vi "LBCB Position Facade.vi"(0 "Data In":T6, 2 "Display State In":T3, 3 "Container State":T5) -> (6 "Data Out":T6, 7 "Display State Out":T3, 8 "Action":T2)   [LabVIEW 2013, in "LBCB Position XC.xctl"]
uses:
  LBCB Position XC.xctl
  lib/Data Access Objects/Metadata/LBCB Position.ctl
  LBCB Position Data.ctl
  <vilib>/_xctls/Container State.ctl
  LBCB Position State.ctl
  lib/Data Access Objects/Application/Number Of LBCBs.ctl
  <vilib>/_xctls/Action.ctl
  <vilib>/_xctls/XControlSupport.lvlib
panel:
  in  "LBCB Position Tab":enum32{"LBCB 1", "LBCB 2"}(tab)
  in  "LBCB Position L1":T1={"Motion Center"=[0.0, 0.0, 0.0], "Transformation Matrix"=[[1.0, 0.0, 0.0, 0.0, 0.0, 0.0], [0.0, 1.0, 0.0, 0.0, 0.0, 0.0], [0.0, 0.0, 1.0, 0.0, 0.0, 0.0], [0.0, 0.0, 0.0, 1.0, 0.0, 0.0], [0.0, 0.0, 0.0, 0.0, 1.0, 0.0], [0.0, 0.0, 0.0, 0.0, 0.0, 1.0]]}
  in  "LBCB Position L2":T1={"Motion Center"=[0.0, 0.0, 0.0], "Transformation Matrix"=[[1.0, 0.0, 0.0, 0.0, 0.0, 0.0], [0.0, 1.0, 0.0, 0.0, 0.0, 0.0], [0.0, 0.0, 1.0, 0.0, 0.0, 0.0], [0.0, 0.0, 0.0, 1.0, 0.0, 0.0], [0.0, 0.0, 0.0, 0.0, 1.0, 0.0], [0.0, 0.0, 0.0, 0.0, 0.0, 1.0]]}
  # "Y"
  # "X"
  # "(inch)"
  # "XLBCB CMD = T-1*XLBCB OM"
  # "Y"
  # "Z"
  # "(inch)"
  # "XOM DISP = T*XLBCB DISP"
  # "Z"
  # "(inch)"
  # "Dx"
  # "Dy"
  # "Dz"
  # "Rx"
  # "Ry"
  # "Rz"
  # "Dx"
  # "Dy"
  # "Dz"
  # "Rx"
  # "Ry"
  # "Rz"
  # "Y"
  # "X"
  # "(inch)"
  # "XLBCB CMD = T-1*XLBCB OM"
  # "Y"
  # "Z"
  # "(inch)"
  # "XOM DISP = T*XLBCB DISP"
  # "Z"
  # "(inch)"
  # "Dx"
  # "Dy"
  # "Dz"
  # "Rx"
  # "Ry"
  # "Rz"
  # "Dx"
  # "Dy"
  # "Dz"
  # "Rx"
  # "Ry"
  # "Rz"
  # "Y"
  # "X"
  # "(inch)"
  # "XLBCB CMD = T-1*XLBCB OM"
  # "Y"
  # "Z"
  # "(inch)"
  # "XOM DISP = T*XLBCB DISP"
  # "Z"
  # "(inch)"
  # "Dx"
  # "Dy"
  # "Dz"
  # "Rx"
  # "Ry"
  # "Rz"
  # "Dx"
  # "Dy"
  # "Dz"
  # "Rx"
  # "Ry"
  # "Rz"
  # "Y"
  # "X"
  # "(inch)"
  # "XLBCB CMD = T-1*XLBCB OM"
  # "Y"
  # "Z"
  # "(inch)"
  # "XOM DISP = T*XLBCB DISP"
  # "Z"
  # "(inch)"
  # "Dx"
  # "Dy"
  # "Dz"
  # "Rx"
  # "Ry"
  # "Rz"
  # "Dx"
  # "Dy"
  # "Dz"
  # "Rx"
  # "Ry"
  # "Rz"
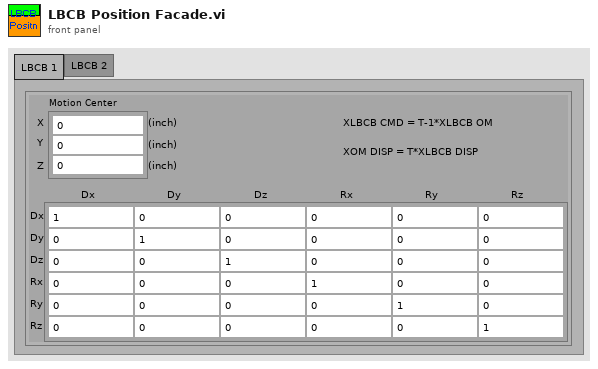
[diagram p1: front panel]
types:
  T1 = typedef "LBCB Position.ctl" = cluster{"Motion Center":dbl[], "Transformation Matrix":dbl[][]}
  T2 = typedef "XControlSupport.lvlib/Action.ctl" = cluster{"Data Changed?":bool, "State Changed?":bool, "Action Name":string}
  T3 = typedef "LBCB Position XC.xctl/LBCB Position State.ctl" = cluster{"Number of LBCBs":T4}
  T4 = typedef "Number Of LBCBs.ctl" = enum16{"1", "2"}
  T5 = typedef "XControlSupport.lvlib/Container State.ctl" = cluster{"Indicator?":bool, "Run Mode?":bool, " Refnum":refnum<vi>}
  T6 = typedef "LBCB Position XC.xctl/LBCB Position Data.ctl" = cluster{"Motion Center":dbl[], "Transformation Matrix":dbl[][]}[]
  T7 = enum8{"Enabled", "Disabled", "Disabled and Grayed Out"}
  T8 = cluster{"Motion Center":dbl[], "Transformation Matrix":dbl[][]}
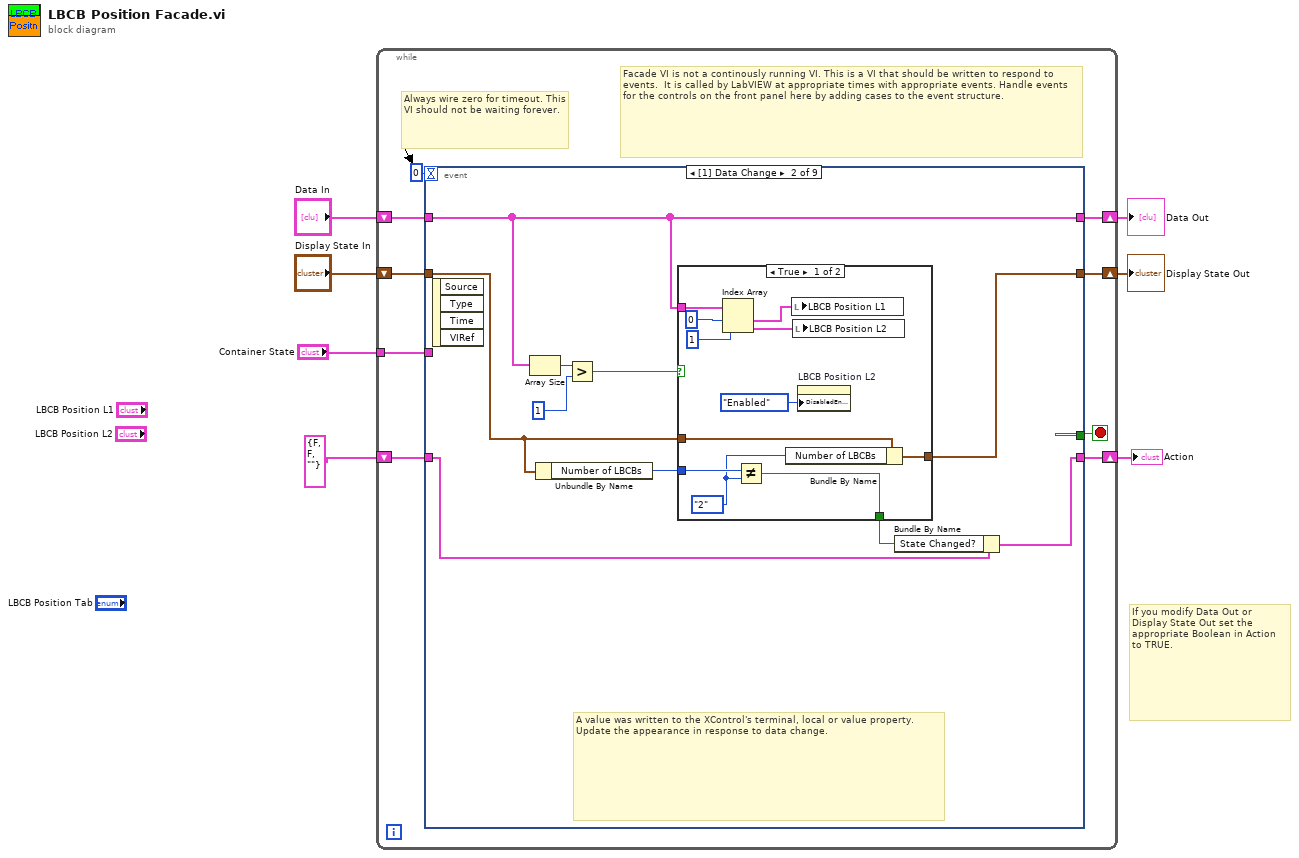
[diagram p0: block diagram]
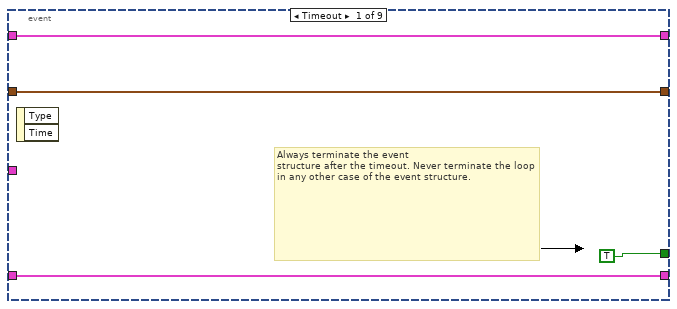
[diagram p2: hidden frame]
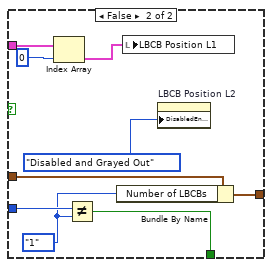
[diagram p3: hidden frame]
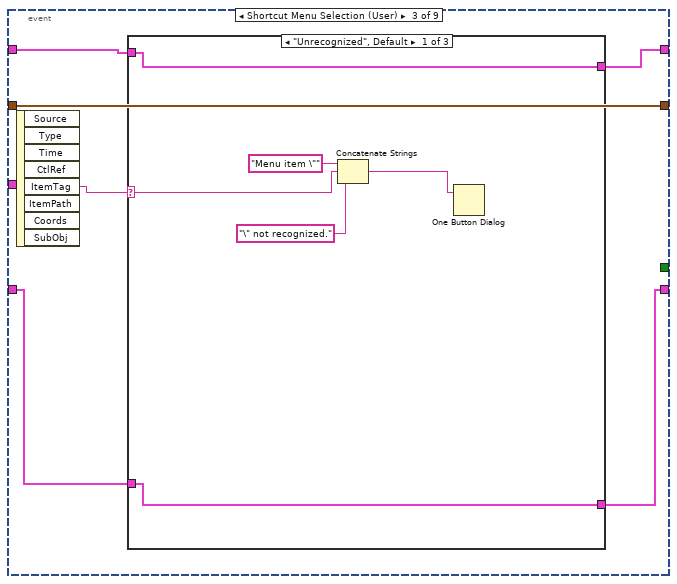
[diagram p4: hidden frame]
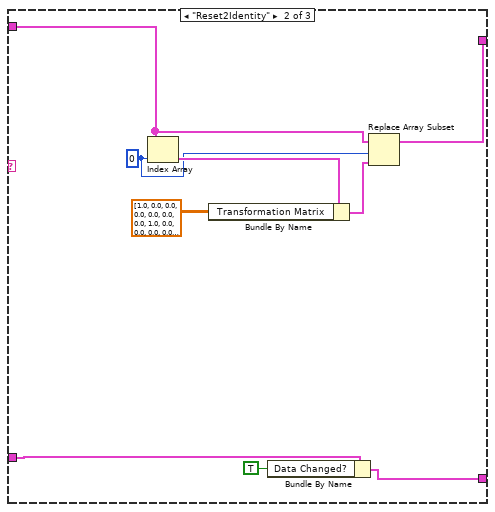
[diagram p5: hidden frame]
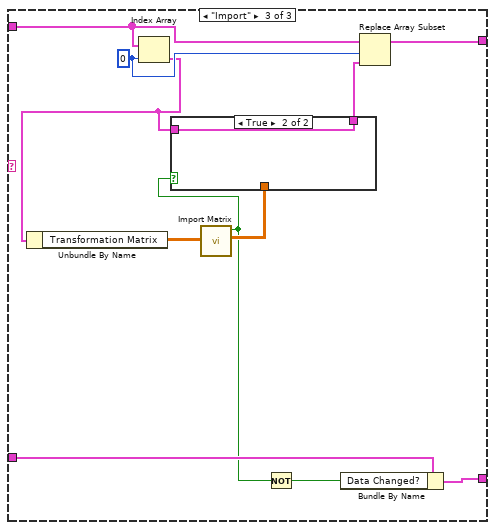
[diagram p6: hidden frame]
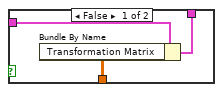
[diagram p7: hidden frame]
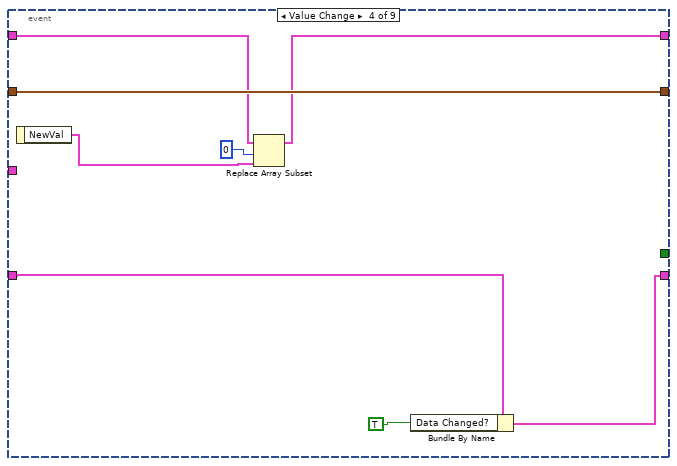
[diagram p8: hidden frame]
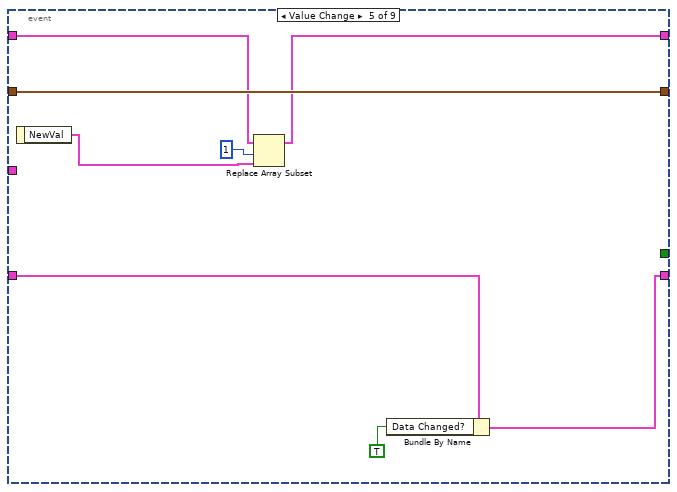
[diagram p9: hidden frame]
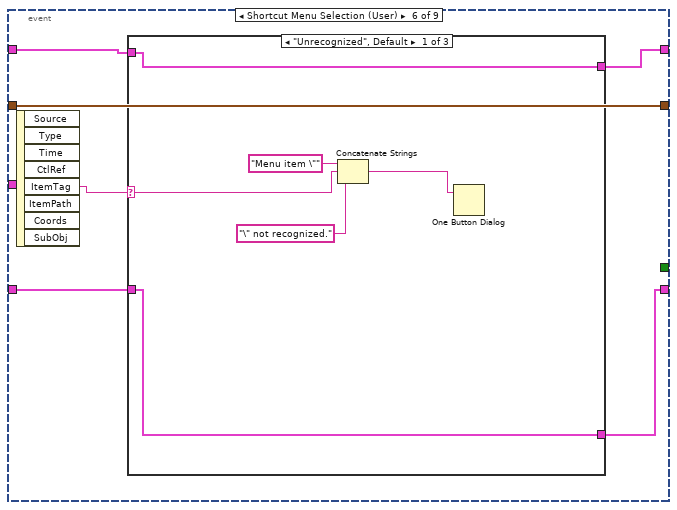
[diagram p10: hidden frame]
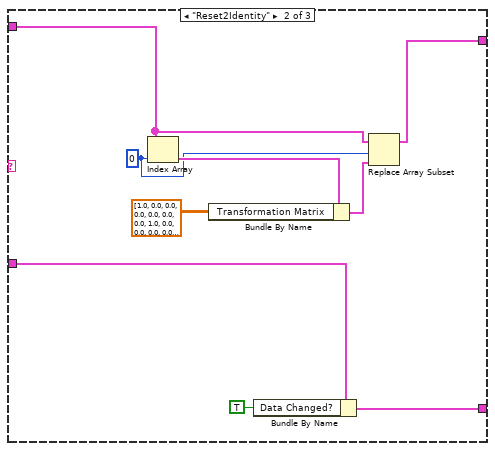
[diagram p11: hidden frame]
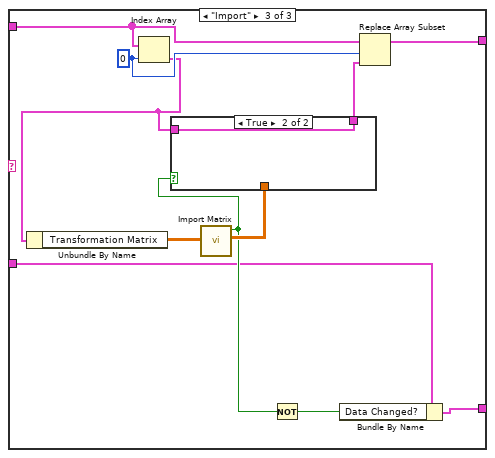
[diagram p12: hidden frame]
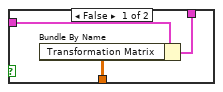
[diagram p13: hidden frame]
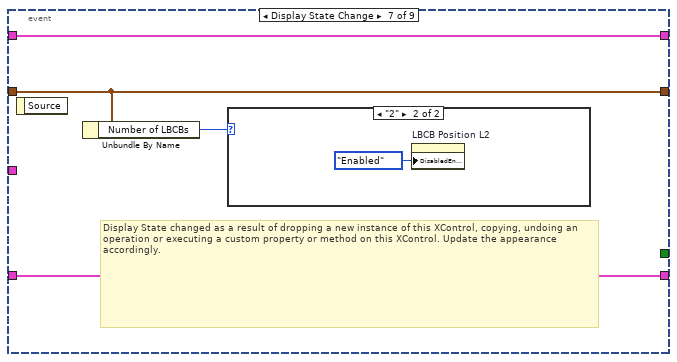
[diagram p14: hidden frame]
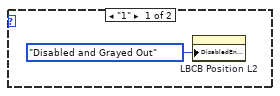
[diagram p15: hidden frame]
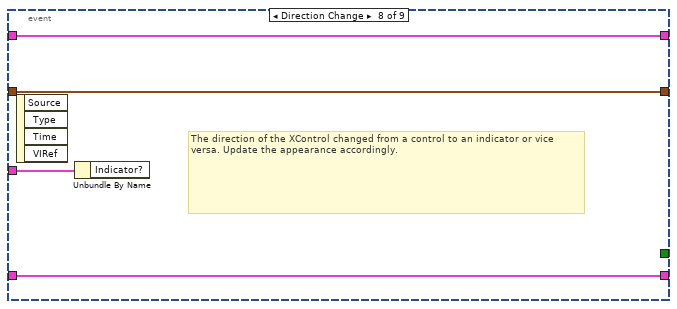
[diagram p16: hidden frame]
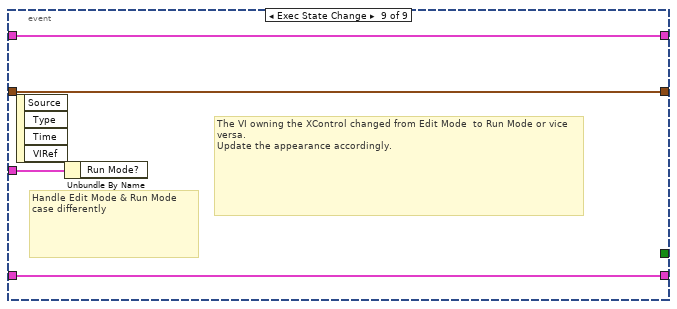
[diagram p17: hidden frame]
diagram:
  # "If you modify Data Out or\nDisplay State Out set the\nappropriate Boolean in Action\nto TRUE."
  n1 = while {
    shift-right: [w15] -> w4
    shift-left: "Display State In" -> [w16]
    tunnel: "Container State" -> [w12]
    shift-right: [w10] -> w7
    shift-left: "Data In" -> [w11]
    shift-right: [w8] -> w2
    shift-left: T2 {"Data Changed?"=FALSE, "State Changed?"=FALSE, "Action Name"=""} ("Action") -> [w9]
    stop <- w14 stop-if-true
    # "Facade VI is not a continously running VI. This is a VI that should be written to respond to events.  It is called by LabVIEW at appropriate times with appropriate events. Handle events for the controls on the front panel here by adding cases to the event structure."
    # "Always wire zero for timeout. This\nVI should not be waiting forever."
    n2 = event shown="[1] Data Change" {
      selector: _ -> [_ _ _ _ _ _ _ _ _]
      dyn-events: _ -> [_ _ _ _ _ _ _ _ _]
      timeout: 0 -> [_ _ _ _ _ _ _ _ _]
      tunnel: w16 -> [w18 w26 w56 w94 w102 w108 w140 w147 w151]
      tunnel: [w18 w21 w56 w94 w102 w108 w140 w147 w151] -> w15
      tunnel: [TRUE _ _ _ _ _ _ _ _] -> w14
      tunnel: w12 -> [_ _ _ _ _ _ _ w148 w152]
      tunnel: w11 -> [w17 w30 w54 w93 w101 w106 w142 w146 w150]
      tunnel: [w17 w30 w53 w90 w98 w105 w142 w146 w150] -> w10
      tunnel: [w19 w22 w51 w88 w95 w103 w141 w145 w149] -> w8
      tunnel: w9 -> [w19 w23 w52 w89 w96 w104 w141 w145 w149]
      event Timeout {
        # "Always terminate the event\nstructure after the timeout. Never terminate the loop in any other case of the event structure."
        n3 = event-data() -> ()  [unwired: 1 in, 2 out]
      }
      event Data Change {
        # "A value was written to the XControl's terminal, local or value property.\nUpdate the appearance in response to data change."
        n4 = event-data() -> ()  [unwired: 1 in, 4 out]
        n5 = Array Size(array=w30) -> (size(s)=w29:i32)
        n6 = Unbundle By Name(w26) -> ("Number of LBCBs"=w25:T4)
        n7 = Greater?(x=w29, y=1) -> (0:w27:bool)
        n8 = case shown="True" w27 {
          tunnel: w30 -> [w41 w50]
          tunnel: w26 -> [w34 w45]
          tunnel: w25 -> [w35 w46]
          tunnel: [w32 w43] -> w24
          tunnel: [w31 w42] -> w21
          frame True {
            w33 = Number_Of_LBCBs."2" ("y")
            n9 = Index Array(array=w41, index #1=0 ("index"), index #2=1 ("index")) -> (element #1=w38:T8, element #2=w37:T8)
            n10 = Not Equal?(x=w35, y=w33) -> (x != y?=w32:bool)
            n11 = Bundle By Name(cluster=w34, "Number of LBCBs"=w33) -> (w31:T3)
            n12 = local write "LBCB Position L1"(w38) -> ()
            n13 = local write "LBCB Position L2"(w37) -> ()
            n14 = property on="LBCB Position L2" class="Clust (strict)"("DisabledEnum"=T7."Enabled" ("Disabled")) -> ()  [unwired: 2 in, 2 out]
          }
          frame False {
            w44 = Number_Of_LBCBs."1" ("y")
            n15 = Index Array(array=w50, index=0) -> (element=w48:T8)
            n16 = Not Equal?(x=w46, y=w44) -> (x != y?=w43:bool)
            n17 = Bundle By Name(cluster=w45, "Number of LBCBs"=w44) -> (w42:T3)
            n18 = local write "LBCB Position L1"(w48) -> ()
            n19 = property on="LBCB Position L2" class="Clust (strict)"("DisabledEnum"=T7."Disabled and Grayed Out" ("Disabled")) -> ()  [unwired: 2 in, 2 out]
          }
        }
        n20 = Bundle By Name(cluster=w23, "State Changed?"=w24) -> (w22:T2)
      }
      event Shortcut Menu Selection (User) {
        n21 = event-data() -> ("ItemTag"=w55:string)  [unwired: 1 in, 7 out]
        n22 = case shown="\"Unrecognized\", Default" w55 {
          selector: w55 -> [w60 _ _]
          tunnel: w54 -> [w58 w68 w81]
          tunnel: [w58 w66 w79] -> w53
          tunnel: w52 -> [w57 w65 w75]
          tunnel: [w57 w64 w74] -> w51
          frame "Unrecognized", Default {
            n23 = Concatenate Strings("Menu item \"" ("string"), w60, "\" not recognized." ("string")) -> (w59:string)
            n24 = One Button Dialog(message=w59) -> ()  [unwired: 1 in, 1 out]
          }
          frame "Reset2Identity" {
            w69 = 0 ("index")
            n25 = Index Array(array=w68, index=w69) -> (element=w71:T8)
            n26 = Bundle By Name(cluster=w71, "Transformation Matrix"=dbl[][] [[1.0, 0.0, 0.0, 0.0, 0.0, 0.0], [0.0, 1.0, 0.0, 0.0, 0.0, 0.0], [0.0, 0.0, 1.0, 0.0, 0.0, 0.0], [0.0, 0.0, 0.0, 1.0, 0.0, 0.0], [0.0, 0.0, 0.0, 0.0, 1.0, 0.0], [0.0, 0.0, 0.0, 0.0, 0.0, 1.0]]) -> (w67:T8)
            n27 = Bundle By Name(cluster=w65, "Data Changed?"=TRUE) -> (w64:T2)
            n28 = Replace Array Subset(array=w68, new element=w67, index=w69) -> (w66:T6)
          }
          frame "Import" {
            w82 = 0 ("index")
            n29 = Index Array(array=w81, index=w82) -> (element=w78:T8)
            n30 = Unbundle By Name(w78) -> ("Transformation Matrix"=w77:dbl[][])
            n31 = call "Import Matrix.vi"("PinPositions In"=w77) -> ("PinPositions Out"=w76:dbl[][], "Canceled"=w73:bool)  [unwired: 9 in]
            n32 = case shown="True" w73 {
              tunnel: [w85 w86] -> w80
              tunnel: w78 -> [w84 w86]
              tunnel: w76 -> [w83 _]
              frame False {
                n33 = Bundle By Name(cluster=w84, "Transformation Matrix"=w83) -> (w85:T8)
              }
              frame True {
              }
            }
            n34 = Not(x=w73) -> (.not. x?=w72:bool)
            n35 = Bundle By Name(cluster=w75, "Data Changed?"=w72) -> (w74:T2)
            n36 = Replace Array Subset(array=w81, new element=w80, index=w82) -> (w79:T6)
          }
        }
      }
      event Value Change {
        n37 = event-data() -> ("NewVal"=w92:T1)  [unwired: 1 in]
        n38 = Replace Array Subset(array=w93, new element=w92, index=0) -> (w90:T6)
        n39 = Bundle By Name(cluster=w89, "Data Changed?"=TRUE) -> (w88:T2)
      }
      event Value Change {
        n40 = event-data() -> ("NewVal"=w100:T1)  [unwired: 1 in]
        n41 = Replace Array Subset(array=w101, new element=w100, index=1) -> (w98:T6)
        n42 = Bundle By Name(cluster=w96, "Data Changed?"=TRUE) -> (w95:T2)
      }
      event Shortcut Menu Selection (User) {
        n43 = event-data() -> ("ItemTag"=w107:string)  [unwired: 1 in, 7 out]
        n44 = case shown="\"Unrecognized\", Default" w107 {
          selector: w107 -> [w112 _ _]
          tunnel: w106 -> [w110 w120 w133]
          tunnel: [w110 w118 w131] -> w105
          tunnel: w104 -> [w109 w117 w125]
          tunnel: [w109 w116 w124] -> w103
          frame "Unrecognized", Default {
            n45 = Concatenate Strings("Menu item \"" ("string"), w112, "\" not recognized." ("string")) -> (w111:string)
            n46 = One Button Dialog(message=w111) -> ()  [unwired: 1 in, 1 out]
          }
          frame "Reset2Identity" {
            w121 = 0 ("index")
            n47 = Index Array(array=w120, index=w121) -> (element=w123:T8)
            n48 = Bundle By Name(cluster=w123, "Transformation Matrix"=dbl[][] [[1.0, 0.0, 0.0, 0.0, 0.0, 0.0], [0.0, 1.0, 0.0, 0.0, 0.0, 0.0], [0.0, 0.0, 1.0, 0.0, 0.0, 0.0], [0.0, 0.0, 0.0, 1.0, 0.0, 0.0], [0.0, 0.0, 0.0, 0.0, 1.0, 0.0], [0.0, 0.0, 0.0, 0.0, 0.0, 1.0]]) -> (w119:T8)
            n49 = Bundle By Name(cluster=w117, "Data Changed?"=TRUE) -> (w116:T2)
            n50 = Replace Array Subset(array=w120, new element=w119, index=w121) -> (w118:T6)
          }
          frame "Import" {
            w134 = 0 ("index")
            n51 = Index Array(array=w133, index=w134) -> (element=w130:T8)
            n52 = Unbundle By Name(w130) -> ("Transformation Matrix"=w129:dbl[][])
            n53 = call "Import Matrix.vi"("PinPositions In"=w129) -> ("PinPositions Out"=w128:dbl[][], "Canceled"=w127:bool)  [unwired: 9 in]
            n54 = case shown="True" w127 {
              tunnel: [w137 w138] -> w132
              tunnel: w130 -> [w136 w138]
              tunnel: w128 -> [w135 _]
              frame False {
                n55 = Bundle By Name(cluster=w136, "Transformation Matrix"=w135) -> (w137:T8)
              }
              frame True {
              }
            }
            n56 = Not(x=w127) -> (.not. x?=w126:bool)
            n57 = Bundle By Name(cluster=w125, "Data Changed?"=w126) -> (w124:T2)
            n58 = Replace Array Subset(array=w133, new element=w132, index=w134) -> (w131:T6)
          }
        }
      }
      event Display State Change {
        # "Display State changed as a result of dropping a new instance of this XControl, copying, undoing an operation or executing a custom property or method on this XControl. Update the appearance accordingly."
        n59 = event-data() -> ()  [unwired: 1 in, 1 out]
        n60 = Unbundle By Name(w140) -> ("Number of LBCBs"=w139:T4)
        n61 = case shown="\"2\"" w139 {
          frame "1" {
            n62 = property on="LBCB Position L2" class="Clust (strict)"("DisabledEnum"=T7."Disabled and Grayed Out" ("Disabled")) -> ()  [unwired: 2 in, 2 out]
          }
          frame "2" {
            n63 = property on="LBCB Position L2" class="Clust (strict)"("DisabledEnum"=T7."Enabled" ("Disabled")) -> ()  [unwired: 2 in, 2 out]
          }
        }
      }
      event Direction Change {
        # "The direction of the XControl changed from a control to an indicator or vice versa. Update the appearance accordingly."
        n64 = event-data() -> ()  [unwired: 1 in, 4 out]
        n65 = Unbundle By Name(w148) -> ()  [unwired: 1 out]
      }
      event Exec State Change {
        # "The VI owning the XControl changed from Edit Mode  to Run Mode or vice versa.\nUpdate the appearance accordingly."
        # "Handle Edit Mode & Run Mode\ncase differently"
        n66 = event-data() -> ()  [unwired: 1 in, 4 out]
        n67 = Unbundle By Name(w152) -> ()  [unwired: 1 out]
      }
    }
  }
  "Display State Out" <- w4
  "Data Out" <- w7
  "Action" <- w2
